vi "BaseGui-Done.vi"(8 "error in":errorcluster) -> (0 "error out":errorcluster)   [LabVIEW 2016]
uses:
  BaseGui.Action.ctl
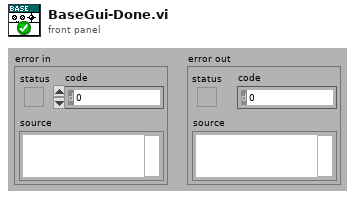
[diagram p1: front panel]
types:
  T1 = typedef "BaseGui.Action.ctl" = enum32{"idle", "constructor", "destructor", "--- BaseGui ---", "Status.Update", "Home.Done"}
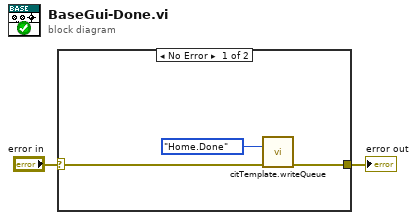
[diagram p0: block diagram]
diagram:
  n1 = case shown="No Error" "error in" {
    selector: "error in" -> [w3 w6]
    tunnel: [w5 w6] -> w1
    frame No Error {
      n2 = call "citTemplate.writeQueue.vi"("event in (if not connected:all statemachine with data event)"=BaseGui.Action."Home.Done" ("Action"), "error in (no error)"=w3) -> ("error out"=w5:errorcluster)  [unwired: 13 in]
    }
    frame Error {
    }
  }
  "error out" <- w1
